vi "gatherPelvicVars.vi"(6 "ViconData":dbl[](array[numeric]), 7 "kconstant":dbl) -> (0 "BoundaryYpelv":dbl[](array[numeric]), 1 "BoundaryXPelv":dbl[](array[numeric]), 2 "pel_cn":dbl[](array[numeric]), 3 "viconData_2":dbl[](array[numeric]), 4 "K constant_pel":dbl, 5 "BoundaryZpelv":dbl[](array[numeric]), 8 "FM --- FF_pel":dbl[](array[numeric]))   [LabVIEW 2017]
panel:
  # "Pelvis Variables for FF"
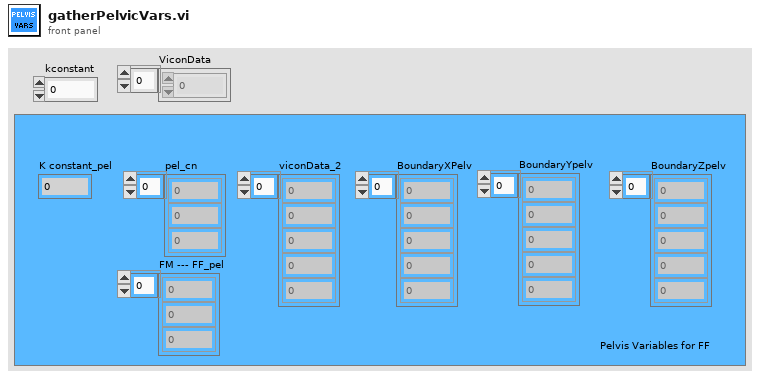
[diagram p1: front panel]
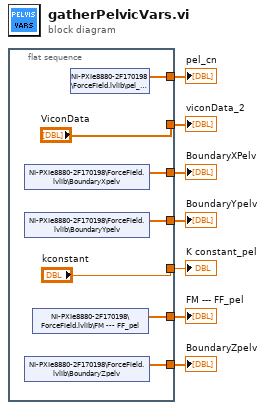
[diagram p0: block diagram]
diagram:
  n1 = flat-sequence {
    tunnel: ["ViconData"] -> w7
    tunnel: [w14] -> w6
    tunnel: [w13] -> w5
    tunnel: [w12] -> w4
    tunnel: ["kconstant"] -> w3
    tunnel: [w11] -> w2
    tunnel: [w10] -> w1
    frame #0 {
      n2 = shared-variable "NI-PXIe8880-2F170198\\ForceField.lvlib\\BoundaryXpelv"() -> (w13:dbl[])  [unwired: 1 in, 1 out]
      n3 = shared-variable "NI-PXIe8880-2F170198\\ForceField.lvlib\\BoundaryYpelv"() -> (w12:dbl[])  [unwired: 1 in, 1 out]
      n4 = shared-variable "NI-PXIe8880-2F170198\\ForceField.lvlib\\BoundaryZpelv"() -> (w10:dbl[])  [unwired: 1 in, 1 out]
      n5 = shared-variable "NI-PXIe8880-2F170198\\ForceField.lvlib\\FM --- FF_pel"() -> (w11:dbl[])  [unwired: 1 in, 1 out]
      n6 = shared-variable "NI-PXIe8880-2F170198\\ForceField.lvlib\\pel_cn"() -> (w14:dbl[])  [unwired: 1 in, 1 out]
    }
  }
  "viconData_2" <- w7
  "pel_cn" <- w6
  "BoundaryXPelv" <- w5
  "BoundaryYpelv" <- w4
  "K constant_pel" <- w3
  "FM --- FF_pel" <- w2
  "BoundaryZpelv" <- w1
